vi "Read dest_endpoint.vi"(8 "error in (no error)":errorcluster, 11 "Zigbee_Send_Msg in":refnum<class "Zigbee_Send_Msg.lvclass">) -> (0 "error out":errorcluster, 2 "dest_endpoint":string, 3 "Zigbee_Send_Msg out":refnum<class "Zigbee_Send_Msg.lvclass">)   [LabVIEW 2020, in "Library Test.lvlib" / "Zigbee_Send_Msg.lvclass"]
uses:
  Zigbee_Send_Msg.lvclass
  Zigbee_Send_Msg.lvclass/Zigbee_Send_Msg.ctl
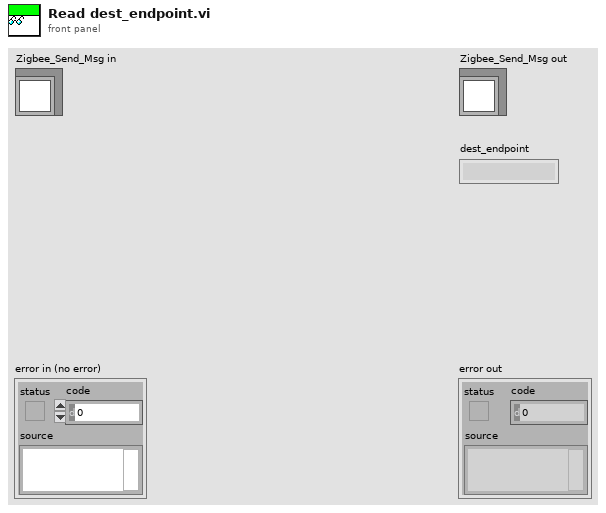
[diagram p1: front panel]
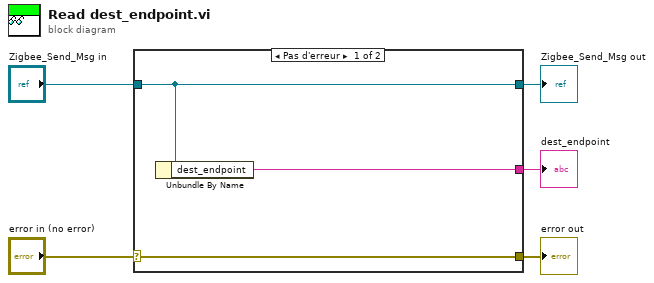
[diagram p0: block diagram]
diagram:
  n1 = case shown="Pas d'erreur" "error in (no error)" {
    selector: "error in (no error)" -> [w8 w9]
    tunnel: [w8 w9] -> w4
    tunnel: [w7 w10] -> w2
    tunnel: "Zigbee_Send_Msg in" -> [w7 w10]
    tunnel: [w6 _] -> w1
    frame No Error {
      n2 = Unbundle By Name(w7) -> ("dest_endpoint"=w6:string)
    }
    frame Error {
    }
  }
  "error out" <- w4
  "Zigbee_Send_Msg out" <- w2
  "dest_endpoint" <- w1
